vi "DCC_set_gain_HV_limit.vi"(6 "Set Gain HV Limit [%]":i16 min=0 max=100, 7 "Limit ID for Connector":i16 min=0 max=1 step=1, 8 "Error In":errorcluster, 10 "Module No":i16, 11 "DLL Path":path) -> (0 "Error Out":errorcluster, 2 "Module No":i16, 3 "DLL Path":path)   [LabVIEW 2019]
doc: "This procedure sets the gain limit in procent for the high voltage output of the specified DCC module by module number. That means the gain HV limit which can be reached by using the \"DCC_set_parameters.vi\".\n\nFurther, the limit ID sets the corresponding connector. Possible values are zero for connector one as well as one for connector three.\n\nAugust 2018\nFrank Quadt & Stefan Smietana\ninfo@becker-hickl.com"
panel:
  # "(c) 2021 Becker & Hickl GmbH\n     All Rights Reserved."
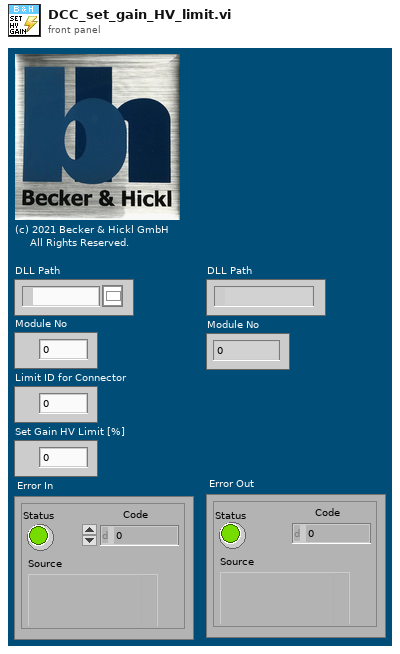
[diagram p1: front panel]
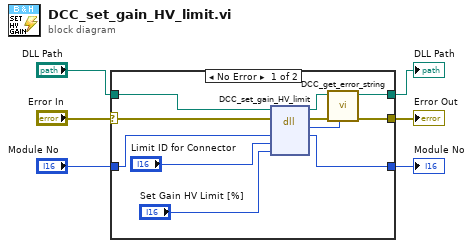
[diagram p0: block diagram]
diagram:
  n1 = case shown="No Error" "Error In" {
    selector: "Error In" -> [w17 w19]
    tunnel: [w9 w19] -> w5
    tunnel: [w10 w20] -> w4
    tunnel: "DLL Path" -> [w15 w20]
    tunnel: "Module No" -> [w14 w18]
    tunnel: [w12 w18] -> w1
    frame No Error {
      n2 = dll-call lib="C:/Program Files/BH/DCC/DLL/dcc32.dll" fn="DCC_set_gain_HV_limit"(path in=w15, error in=w17, "ModuleNo"=w14, "LimitID"="Limit ID for Connector", "Gain"="Set Gain HV Limit [%]") -> (path out=w16:path, error out=w8:errorcluster, "return type"=w7:i16, "ModuleNo"=w12:i16)  [unwired: 3 in]
      n3 = call "DCC_get_error_string.vi"("Error ID"=w7, "Error In"=w8, "DLL Path"=w16) -> ("Error Out"=w9:errorcluster, "DLL Path"=w10:path)  [unwired: 6 in, 1 out]
    }
    frame Error {
    }
  }
  "Error Out" <- w5
  "DLL Path" <- w4
  "Module No" <- w1
